vi "general_control_from_CSV.vi"() -> ()   [LabVIEW 2021]
uses:
  <vilib>/DAQmx/create/channels.llb/DAQmx Create Channel (AO-Voltage-Basic).vi
  <vilib>/DAQmx/write.llb/DAQmx Write (Analog 1D DBL NChan 1Samp).vi
  <vilib>/Utility/file.llb/Read Delimited Spreadsheet (DBL).vi
panel:
  out "Cycles Completed":i32
  out "561 (Automated)":dbl
  out "Phase II Iterations":i32
  in  "TickLength":u32
  in  "Y1 (-10-10V)":dbl
  in  "X1 (-10-10V)":dbl
  in  "514 (0-10v)":dbl
  in  "488 (0-10v)":dbl
  in  "445 (0-10v)":dbl
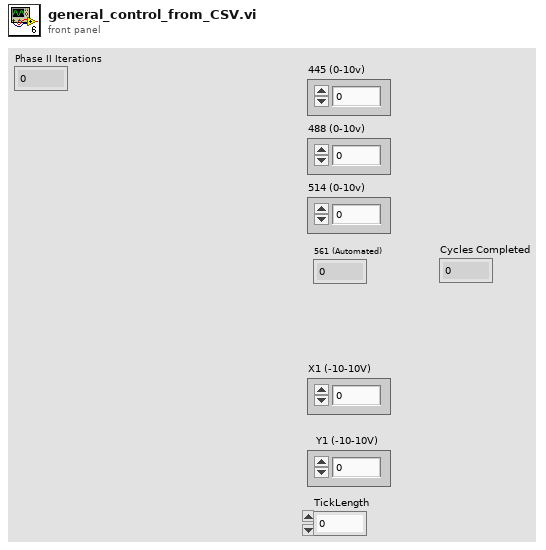
[diagram p1: front panel]
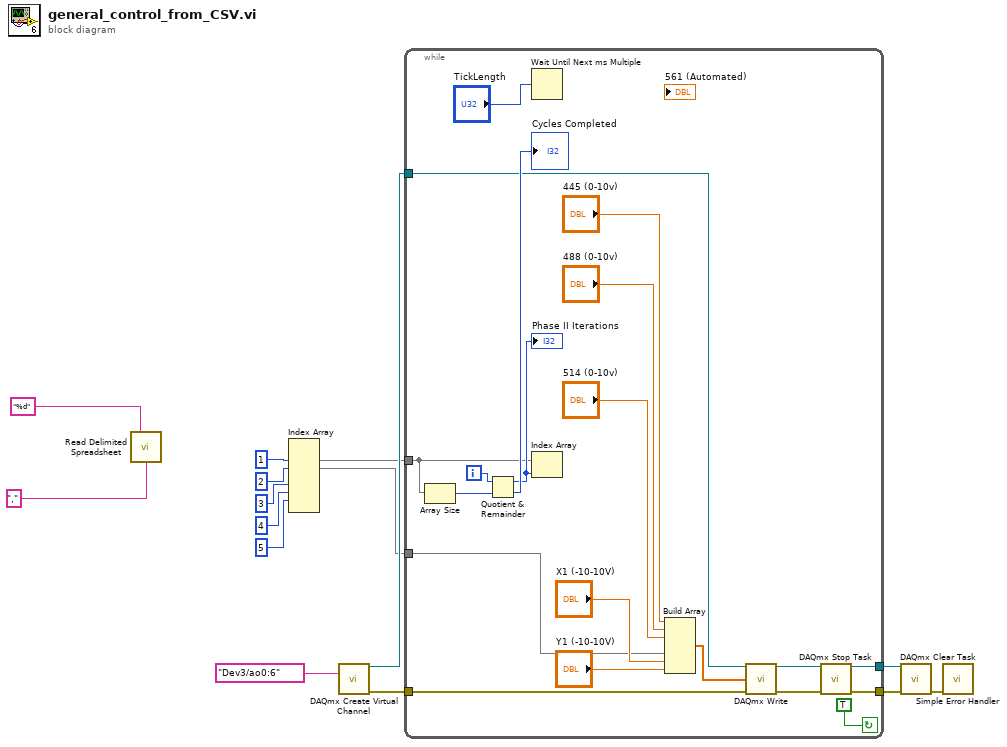
[diagram p0: block diagram]
diagram:
  n1 = call-poly <vilib>:"Read Delimited Spreadsheet.vi"("format (%.3f)"="%d", "delimiter (\\t)"=",") -> ()  [unwired: 8 in, 6 out]
  n2 = Index Array(index #1=1, index #2=2, index #4=3, index #5=4, index #6=5) -> (element #1=w6, element #2=w1)  [unwired: 3 in, 5 out]
  n3 = call-poly <vilib>:"DAQmx Create Virtual Channel.vi"("physical channels"=tag "Dev3/ao0:6") -> ("task out"=w9:refnum<k21>, "error out"=w8:errorcluster)  [unwired: 13 in]
  n4 = while {
    tunnel: [w26] -> w13
    tunnel: [w27] -> w12
    tunnel: w6 -> [w17]
    tunnel: w9 -> [w21]
    tunnel: w8 -> [w20]
    tunnel: w1 -> [w16]
    i -> [w25]
    stop <- TRUE continue-if-true
    n5 = Array Size(array=w17) -> (size(s)=w24:i32)
    n6 = Quotient & Remainder(x=w25, y=w24) -> (x-y*floor(x/y)=w22:i32, floor(x/y)=→"Cycles Completed":i32)
    "Phase II Iterations" <- w22
    n7 = Wait Until Next ms Multiple(millisecond multiple="TickLength") -> ()  [unwired: 1 out]
    n8 = Index Array "Index Array"(array=w17, index=w22) -> ()  [unwired: 1 out]
    n9 = Build Array("445 (0-10v)", "488 (0-10v)", "514 (0-10v)", w16, "X1 (-10-10V)", "Y1 (-10-10V)") -> (w35:dbl[])  [unwired: 1 in]
    n10 = call-poly <vilib>:"DAQmx Write.vi"("task/channels in"=w21, "data"=w35, "error in"=w20) -> ("task out"=w19:refnum<k21>, "error out"=w18:errorcluster)  [unwired: 10 in, 1 out]
    n11 = call <vilib>:"DAQmx Stop Task.vi"("task/channels in"=w19, "error in"=w18) -> ("task out"=w26:refnum<k21>, "error out"=w27:errorcluster)  [unwired: 12 in]
  }
  n12 = call <vilib>:"DAQmx Clear Task.vi"("task in"=w13, "error in"=w12) -> ("error out"=w15:errorcluster)  [unwired: 13 in]
  n13 = call <vilib>:"Simple Error Handler.vi"("error in (no error)"=w15) -> ()  [unwired: 4 in, 5 out]
